vi "Initialize Bus Monitor.vi"(8 "error in (no error)":errorcluster, 11 "ListboxBusMonitor In":refnum<class "ListboxBusMonitor.lvclass">) -> (0 "error out":errorcluster, 3 "ListboxBusMonitor Out":refnum<class "ListboxBusMonitor.lvclass">)   [LabVIEW 2019, in "ListboxBusMonitor.lvlib" / "ListboxBusMonitor.lvclass"]
uses:
  <vilib>/gpm_packages/@cs/BusMonitor/ListboxBusMonitor/ListboxBusMonitor/ListboxBusMonitor.lvclass
  <vilib>/gpm_packages/@cs/BusMonitor/ListboxBusMonitor/ListboxBusMonitor/ListboxBusMonitor.lvclass/ListboxBusMonitor.ctl
  <vilib>/gpm_packages/@cs/BusMonitor/ListboxBusMonitor/ListboxBusMonitorPanel/ListboxBusMonitorPanel.lvclass/ListboxBusMonitorPanel.ctl
  <vilib>/gpm_packages/@cs/BusMonitor/ListboxBusMonitor/ListboxBusMonitorPanel/ListboxBusMonitorPanel.lvclass
  C:/Program Files/National Instruments/LabVIEW 2019/vi.lib/ActorFramework/Actor/Actor.lvclass
  <vilib>/ActorFramework/Actor/Actor.lvclass
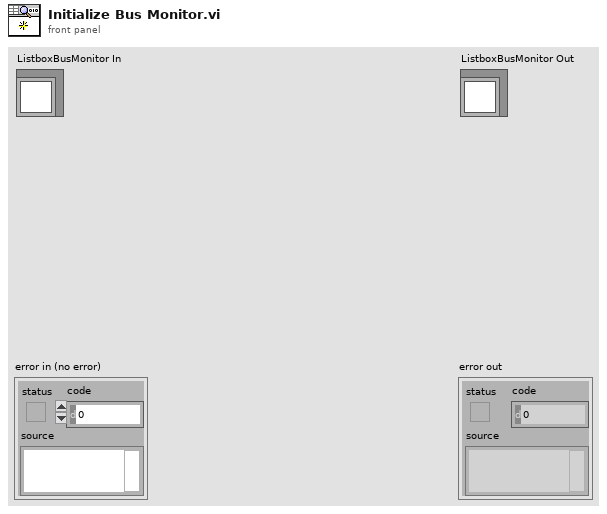
[diagram p1: front panel]
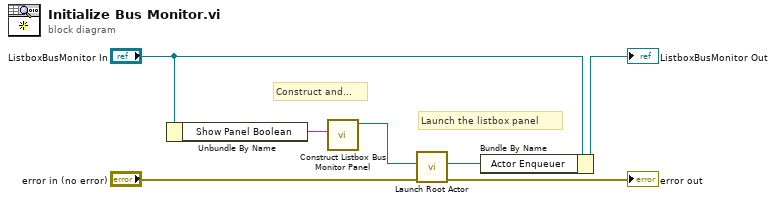
[diagram p0: block diagram]
diagram:
  # "Construct and..."
  # "Launch the listbox panel"
  n1 = Unbundle By Name("ListboxBusMonitor In") -> ("Show Panel Boolean"=w1:string)
  n2 = call <vilib>:"Construct Listbox Bus Monitor Panel.vi"("Show Panel Boolean"=w1) -> ("ListboxBusMonitorPanel out"=w3:refnum<class "ListboxBusMonitorPanel.lvclass">)  [unwired: 10 in]
  n3 = call <vilib>:"Launch Root Actor.vi"("error in (no error)"="error in (no error)", "Actor"=w3) -> ("error out"=→"error out":errorcluster, "Actor's Enqueuer"=w4:refnum<class "Message Enqueuer.lvclass">)  [unwired: 8 in]
  n4 = Bundle By Name(cluster="ListboxBusMonitor In", "Actor Enqueuer"=w4) -> (→"ListboxBusMonitor Out":refnum<class "ListboxBusMonitor.lvclass">)
